vi "oa_Convert EU to Volt (Even Angle, N Channels).vi"(8 "error in (no error)":errorcluster, 10 "even angle channel info":T4[](array[typedef]) {"channel info"."pregain" format="%.2f"; "channel info"."weighting filter" items=["Linear", "A-weighting", "B-weighting", "C-weighting", "ITU-R 468-4", "Dolby", "CCITT", "C-message", "Wb", "Wc", "Wd", "We", "Wf", "Wh", "Wj", "Wk", "Wm", "AES17 20 kHz lowpass", "AES17 40 kHz lowpass", "AES17 20 kHz highpass", "AES17 40 kHz highpass"]; "channel info"."dB reference" format="%^.1e"; "channel info"."engineering units" items=["custom..."=0, "V"=1, "A"=21, "C"=30, "pC"=31, "s"=32, "-"=29, "Pa"=2, "N"=20, "g"=3, "m/s^2"=4, "m/s"=5, "m"=6, "mm/s"=12, "mm"=13, "micron/s"=14, "micron"=15, "in/s^2"=7, "in/s"=8, "in"=9, "mil/s"=10, "mil"=11, "rad/s^2"=16, "rad/s"=17, "rad"=18, "deg/s^2"=26, "deg/s"=27, "deg"=28, "RPM"=22, "cycle/s^2"=23, "Hz"=24, "cycle"=25, "strain"=19]; "channel info"."sensor sensitivity" format="%#_5f"}, 11 "even angle signals":cluster{"r0":dbl, "dr":dbl, "Y":dbl[]}[](array[cluster]) {"r0" format="%.2p"; "dr" format="%.2p"; "Y" format="%.2f"}) -> (0 "error out":errorcluster, 2 "channel info":T1[](array[typedef]) {"pregain" format="%.2f"; "weighting filter" items=["Linear", "A-weighting", "B-weighting", "C-weighting", "ITU-R 468-4", "Dolby", "CCITT", "C-message", "Wb", "Wc", "Wd", "We", "Wf", "Wh", "Wj", "Wk", "Wm", "AES17 20 kHz lowpass", "AES17 40 kHz lowpass", "AES17 20 kHz highpass", "AES17 40 kHz highpass"]; "dB reference" format="%^.1e"; "engineering units" items=["custom..."=0, "V"=1, "A"=21, "C"=30, "pC"=31, "s"=32, "-"=29, "Pa"=2, "N"=20, "g"=3, "m/s^2"=4, "m/s"=5, "m"=6, "mm/s"=12, "mm"=13, "micron/s"=14, "micron"=15, "in/s^2"=7, "in/s"=8, "in"=9, "mil/s"=10, "mil"=11, "rad/s^2"=16, "rad/s"=17, "rad"=18, "deg/s^2"=26, "deg/s"=27, "deg"=28, "RPM"=22, "cycle/s^2"=23, "Hz"=24, "cycle"=25, "strain"=19]; "sensor sensitivity" format="%#_5f"}, 3 "even angle signals":cluster{"r0":dbl, "dr":dbl, "Y":dbl[]}[](array[cluster]) {"r0" format="%.2p"; "dr" format="%.2p"; "Y" format="%.2f"})   [LabVIEW 2017, in "SoundVib_RefDataProcess.lvlib"]
uses:
  <vilib>/addons/Sound and Vibration/Order Analysis/Referece Data Processing/SoundVib_RefDataProcess.lvlib
  <vilib>/addons/_NISVFA/_Shared subVIs/Controls/svc_Resampled Channel Info.ctl
  <vilib>/addons/_NISVFA/_Shared subVIs/Controls/svc_Channel Info.ctl
  <vilib>/addons/_NISVFA/_Shared subVIs/Controls/svc_Engineering Units Text Ring.ctl
  <vilib>/addons/_NISVFA/_Shared subVIs/Controls/svc_Weighting Filter Text Ring.ctl
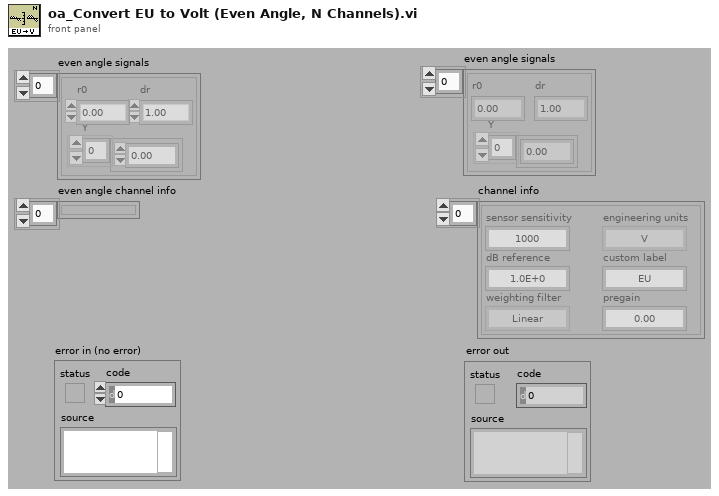
[diagram p1: front panel]
types:
  T1 = typedef "svc_Channel Info.ctl" = cluster{"sensor sensitivity":dbl, "engineering units":T2, "dB reference":dbl, "custom label":string, "weighting filter":T3, "pregain":dbl}
  T2 = typedef "svc_Engineering Units Text Ring.ctl" = u16
  T3 = typedef "svc_Weighting Filter Text Ring.ctl" = u16
  T4 = typedef "svc_Resampled Channel Info.ctl" = cluster{"channel name":string, "description":string, " channel info":T1}
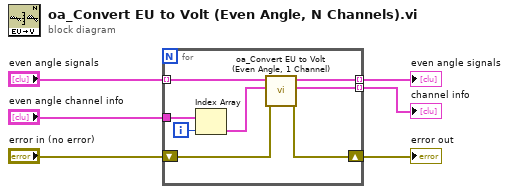
[diagram p0: block diagram]
diagram:
  n1 = for {
    tunnel: "even angle signals" -> [w12] mode=indexing
    tunnel: "even angle channel info" -> [w14]
    tunnel: [w10] -> w4 mode=indexing
    tunnel: [w9] -> w3 mode=indexing
    shift-right: [w7] -> w1
    shift-left: "error in (no error)" -> [w8]
    i -> [w13]
    n2 = Index Array(array=w14, index=w13) -> (element=w11:T4)
    n3 = call <vilib>:"oa_Convert EU to Volt (Even Angle, 1 Channel).vi"("error in (no error)"=w8, "even angle channel info"=w11, "even angle signal"=w12) -> ("error out"=w7:errorcluster, "channel info"=w9:T1, "even angle signal"=w10:cluster{"r0":dbl, "dr":dbl, "Y":dbl[]})  [unwired: 6 in]
  }
  "error out" <- w1
  "even angle signals" <- w4
  "channel info" <- w3
